vi "UpdateTagsToErrorUX.vi"(8 "error in (no error)":errorcluster, 10 "Tag Map":map{string, string}(c390), 11 "ErrorUX In":T1) -> (0 "error out":errorcluster, 3 "ErrorUX Out":T1)   [LabVIEW 2019, in "LabErrorUX.lvclass"]
uses:
  LabErrorUX.lvclass
  Typedefs/ErrorUX.ctl
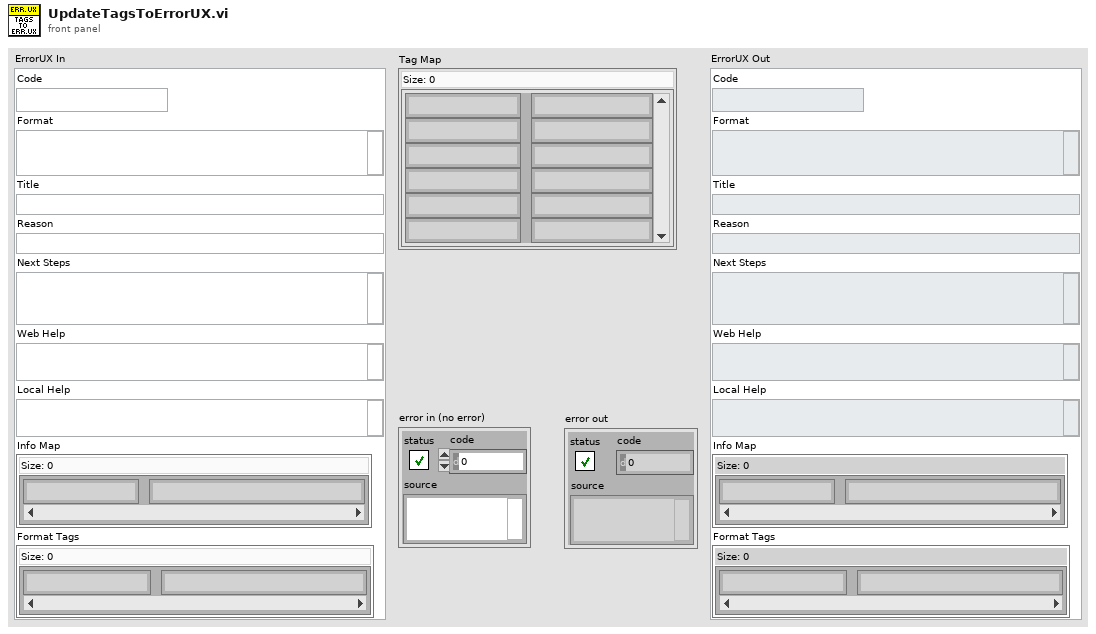
[diagram p1: front panel]
types:
  T1 = typedef "LabErrorUX.lvclass/ErrorUX.ctl" = cluster{"Code":string, "Format":string, "Title":string, "Reason":string, "Next Steps":string, "Web Help":string, "Local Help":string, "Info Map":map{string, string}, "Format Tags":map{string, string}}
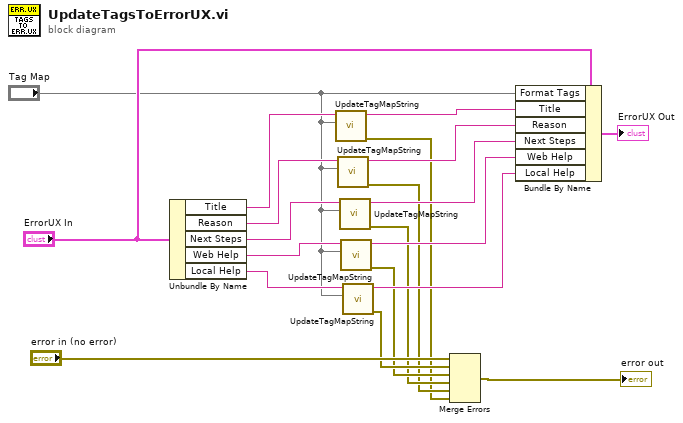
[diagram p0: block diagram]
diagram:
  n1 = Unbundle By Name("ErrorUX In") -> ("Title"=w20:string, "Reason"=w19:string, "Next Steps"=w18:string, "Web Help"=w17:string, "Local Help"=w16:string)
  n2 = call "UpdateTagMapString.vi"("Tag Map"="Tag Map", "Input String"=w20) -> ("error out"=w3:errorcluster, "Output String"=w14:string)  [unwired: 8 in]
  n3 = call "UpdateTagMapString.vi"("Tag Map"="Tag Map", "Input String"=w19) -> ("error out"=w4:errorcluster, "Output String"=w13:string)  [unwired: 8 in]
  n4 = call "UpdateTagMapString.vi"("Tag Map"="Tag Map", "Input String"=w18) -> ("error out"=w5:errorcluster, "Output String"=w12:string)  [unwired: 8 in]
  n5 = call "UpdateTagMapString.vi"("Tag Map"="Tag Map", "Input String"=w17) -> ("error out"=w6:errorcluster, "Output String"=w11:string)  [unwired: 8 in]
  n6 = call "UpdateTagMapString.vi"("Tag Map"="Tag Map", "Input String"=w16) -> ("error out"=w7:errorcluster, "Output String"=w10:string)  [unwired: 8 in]
  n7 = Merge Errors("error in (no error)", w7, w6, w5, w4, w3) -> (→"error out":errorcluster)
  n8 = Bundle By Name(cluster="ErrorUX In", "Format Tags"="Tag Map", "Title"=w14, "Reason"=w13, "Next Steps"=w12, "Web Help"=w11, "Local Help"=w10) -> (→"ErrorUX Out":T1)
